vi "子VI的创建与调用.vi"() -> ()   [LabVIEW 2018]
panel:
  out "方波":dbl[](graph)
  out "锯齿波":dbl[](graph)
  in  "幅值 3":dbl(knob) scale=0.0..10.0
  in  "幅值 2":dbl(knob) scale=0.0..10.0
  in  "幅值1":dbl(knob) scale=0.0..10.0
  out "三角波":dbl[](graph)
  # "编写一个产生三角波、锯齿波和方波的子VI，波形的幅度可调，利用VI调用该子VI，同时，\n在VI中对波形进行整体向上平移2个单位再显示出来。"
  # "20174080221\n王靖\n电子二班"
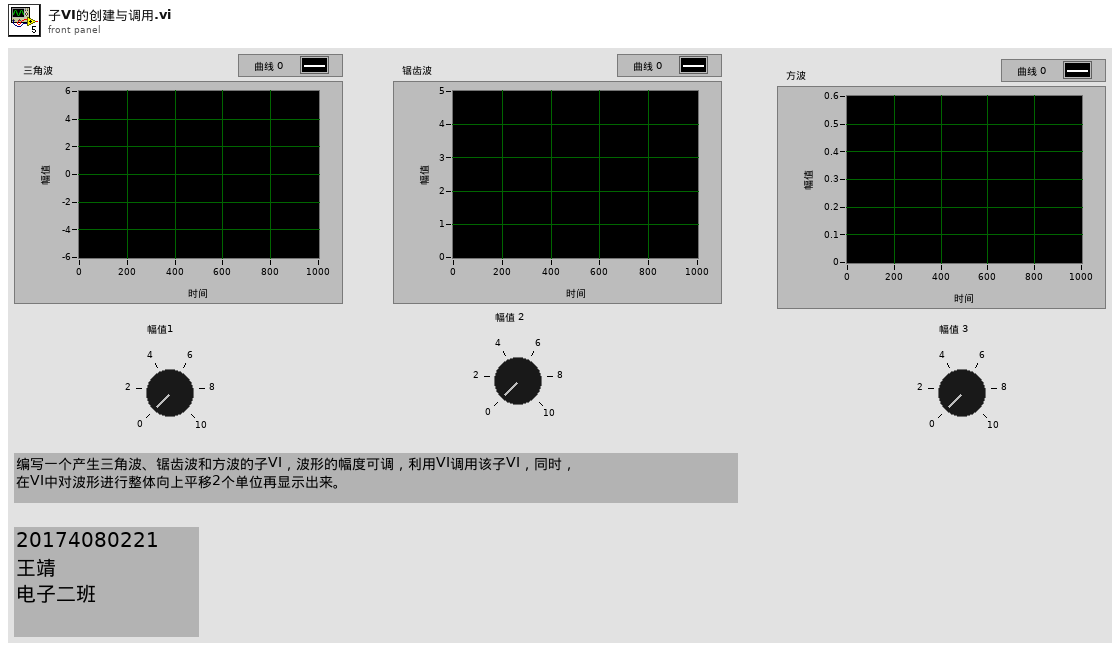
[diagram p1: front panel]
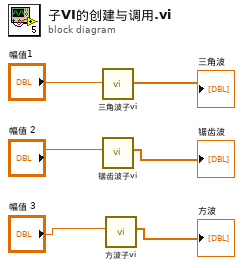
[diagram p0: block diagram]
diagram:
  n1 = call "三角波子vi.vi"("幅值"="幅值1") -> ("数组"=→"三角波":dbl[])  [unwired: 10 in]
  n2 = call "锯齿波子vi.vi"("幅值"="幅值 2") -> ("数组"=→"锯齿波":dbl[])  [unwired: 10 in]
  n3 = call "方波子vi.vi"("幅值"="幅值 3") -> ("数组"=→"方波":dbl[])  [unwired: 10 in]
